vi "PCP HV on OK.vi"(1 "Action(GET)":enum16{"GET", "SET"}(ring), 7 "PCP HV on OK":bool, 9 "Telemetry Started":bool, 11 "error in (no error)":errorcluster, 12 "HV Active":bool) -> (8 "PCP cHV on OKout":bool, 10 "Telemetry Started out":bool, 14 "HV Active out":bool, 15 "error out":errorcluster)   [LabVIEW 2011]
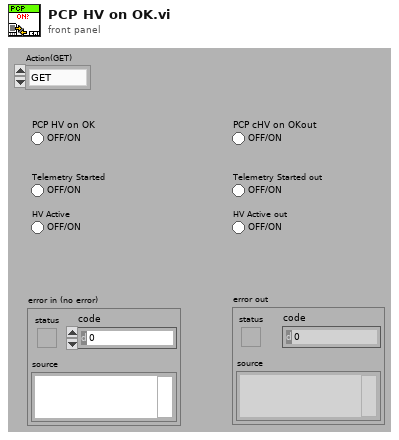
[diagram p1: front panel]
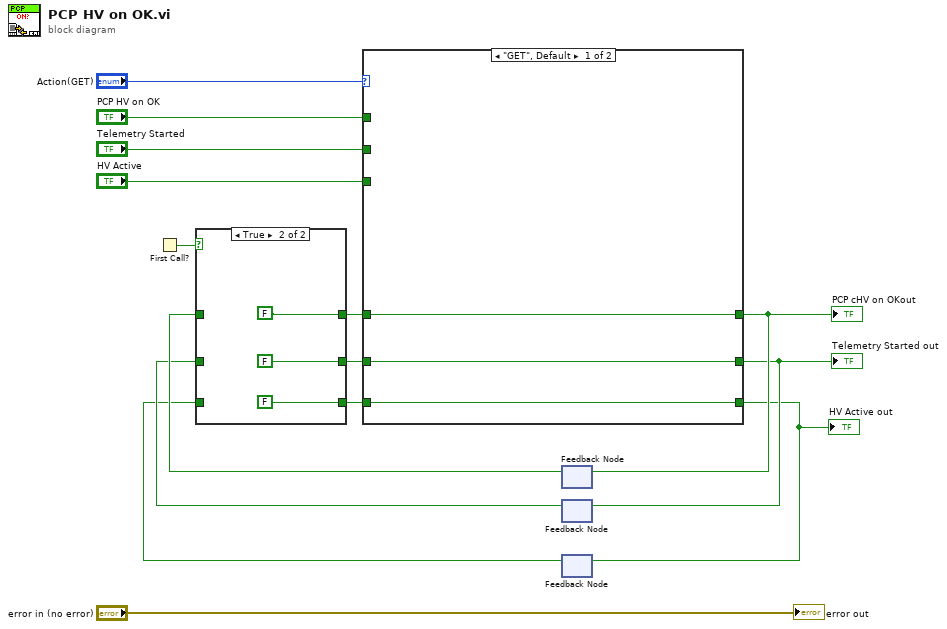
[diagram p0: block diagram]
diagram:
  n1 = First Call?() -> (First Call?: T/F=w12:bool)
  n2 = feedback #1() -> (w13:bool)  [unwired: 1 in]
  n3 = feedback #2() -> (w5:bool)  [unwired: 1 in]
  n4 = feedback #3() -> (w1:bool)  [unwired: 1 in]
  n5 = case shown="True" w12 {
    tunnel: w13 -> [w18 _]
    tunnel: [w18 FALSE ("Tool connected")] -> w10
    tunnel: [w17 FALSE ("Tool connected")] -> w7
    tunnel: w5 -> [w17 _]
    tunnel: [w16 FALSE ("HV Active")] -> w3
    tunnel: w1 -> [w16 _]
    frame False {
    }
    frame True {
    }
  }
  n6 = case shown="\"GET\", Default" "Action(GET)" {
    tunnel: [w24 w27] -> w11
    tunnel: w10 -> [w24 _]
    tunnel: "PCP HV on OK" -> [_ w27]
    tunnel: "Telemetry Started" -> [_ w26]
    tunnel: [w23 w26] -> w6
    tunnel: w7 -> [w23 _]
    tunnel: "HV Active" -> [_ w25]
    tunnel: [w22 w25] -> w2
    tunnel: w3 -> [w22 _]
    frame "GET", Default {
    }
    frame "SET" {
    }
  }
  "PCP cHV on OKout" <- w11
  "Telemetry Started out" <- w6
  "HV Active out" <- w2
  n7 = feedback-in #1(w11) -> ()
  n8 = feedback-in #2(w6) -> ()
  n9 = feedback-in #3(w2) -> ()
  "error out" <- "error in (no error)"
